vi "X-Light V2 Parse Positions.vi"(0 "Recived Reply":string, 11 "Error In":errorcluster) -> (4 "Filter Wheel":i32, 6 "Dichroic":i32, 8 "Disk":i32, 10 "Disk On":bool, 15 "Error Out":errorcluster)   [LabVIEW 2020]
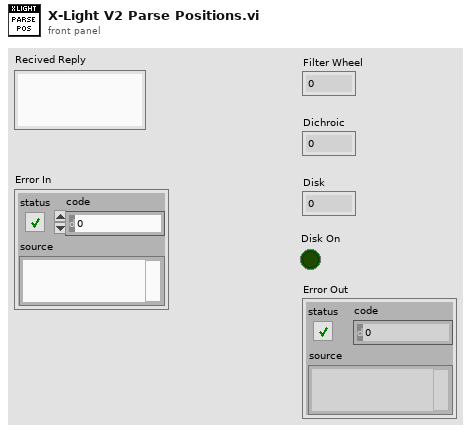
[diagram p1: front panel]
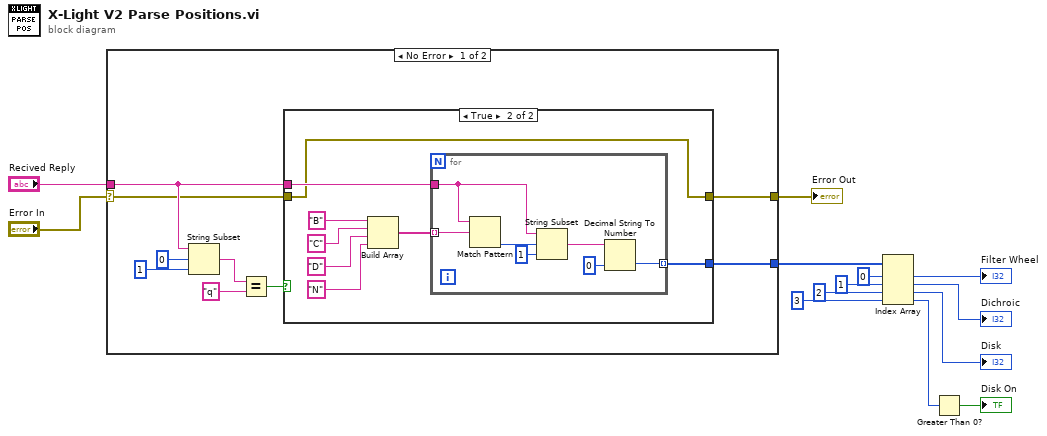
[diagram p0: block diagram]
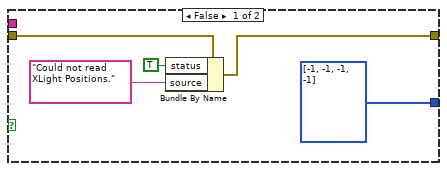
[diagram p2: hidden frame]
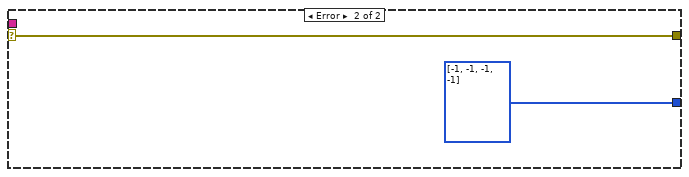
[diagram p3: hidden frame]
diagram:
  n1 = case shown="No Error" "Error In" {
    selector: "Error In" -> [w16 w43]
    tunnel: "Recived Reply" -> [w19 _]
    tunnel: [w17 i32[] [-1, -1, -1, -1]] -> w13
    tunnel: [w15 w43] -> w5
    frame No Error {
      n2 = String Subset(string=w19, offset (0)=0, length (rest)=1 ("length (rest)")) -> (substring=w20:string)
      n3 = Equal?(x=w20, y="q") -> (x = y?=w18:bool)
      n4 = case shown="True" w18 {
        tunnel: w19 -> [_ w35]
        tunnel: [i32[] [-1, -1, -1, -1] w29] -> w17
        tunnel: w16 -> [w26 w28]
        tunnel: [w23 w28] -> w15
        frame False {
          n5 = Bundle By Name(cluster=w26, "status"=TRUE, "source"="Could not read XLight Positions.") -> (w23:errorcluster)
        }
        frame True {
          n6 = Build Array("B" ("regular expression"), "C" ("regular expression"), "D" ("regular expression"), "N" ("regular expression")) -> (w30:string[])
          n7 = for {
            tunnel: w35 -> [w40]
            tunnel: w30 -> [w39] mode=indexing
            tunnel: [w36] -> w29 mode=indexing
            n8 = Match Pattern(string=w40, regular expression=w39) -> (offset past match=w42:i32)  [unwired: 1 in, 3 out]
            n9 = String Subset(string=w40, offset (0)=w42, length (rest)=1 ("length (rest)")) -> (substring=w38:string)
            n10 = Decimal String To Number(string=w38, default (0L)=0 ("default (0 I32)")) -> (number=w36:i32)  [unwired: 1 in, 1 out]
          }
        }
      }
    }
    frame Error {
    }
  }
  "Error Out" <- w5
  n11 = Index Array(array=w13, index #1=0 ("index"), index #2=1 ("index"), index #3=2 ("index"), index #4=3 ("index")) -> (element #1=→"Filter Wheel":i32, element #2=→"Dichroic":i32, element #3=→"Disk":i32, element #4=w8:i32)
  n12 = Greater Than 0?(x=w8) -> (x > 0?=→"Disk On":bool)
